vi "Wait.vi"(8 "Error In":errorcluster, 9 "timeout in ms (-1)":i32=-1, 11 "Init Waiter in":refnum<class "Init Waiter.lvclass">) -> (0 "Error Out":errorcluster, 1 "timed out?":bool)   [LabVIEW 2020, in "Panel.lvlib" / "Init Waiter.lvclass"]
doc: "Waits for the Panel to be initialized.\n<B>Init Waiter In:</B> Init Waiter to wait on\n<B>timeout in ms (-1):</B> Time to wait before timing out.\n<B>Error In:</B> Describes error conditions that occur before this node runs.\n\n<B>timed out?:</B> Indicates if the operation timed out.\n<B>Error Out:</B> Contains error information.\n----\nPlease see the following web address for additional documentation and tutorial information:\nhttp://www.mooregoodideas.com/mgi-panel-manager/\n\nAuthor: Derek Trepanier\n\nCopyright (c) 2018, Moore Good Ideas, Inc.\n\nAll rights reserved.\n\nRedistribution and use in source and binary forms, with or without modification, are permitted provided that the following conditions are met:\n\n * Redistributions of source code must retain the above copyright notice, this list of conditions and the following disclaimer.\n * Redistributions in binary form must reproduce the above copyright notice, this list of conditions and the following disclaimer in the documentation and/or other materials provided with the distribution.\n * Neither the name of Moore Good Ideas, Inc. nor the names of its contributors may be used to endorse or promote products derived from this software without specific prior written permission.\n\nTHIS SOFTWARE IS PROVIDED BY THE COPYRIGHT HOLDERS AND CONTRIBUTORS \"AS IS\" AND ANY EXPRESS OR IMPLIED WARRANTIES, INCLUDING, BUT NOT LIMITED TO, THE IMPLIED WARRANTIES OF MERCHANTABILITY AND FITNESS FOR A PARTICULAR PURPOSE ARE DISCLAIMED. IN NO EVENT SHALL THE COPYRIGHT OWNER OR CONTRIBUTORS BE LIABLE FOR ANY DIRECT, INDIRECT, INCIDENTAL, SPECIAL, EXEMPLARY, OR CONSEQUENTIAL DAMAGES (INCLUDING, BUT NOT LIMITED TO, PROCUREMENT OF SUBSTITUTE GOODS OR SERVICES; LOSS OF USE, DATA, OR PROFITS; OR BUSINESS INTERRUPTION) HOWEVER CAUSED AND ON ANY THEORY OF LIABILITY, WHETHER IN CONTRACT, STRICT LIABILITY, OR TORT (INCLUDING NEGLIGENCE OR OTHERWISE) ARISING IN ANY WAY OUT OF THE USE OF THIS SOFTWARE, EVEN IF ADVISED OF THE POSSIBILITY OF SUCH DAMAGE."
uses:
  <vilib>/MGI/Panel Manager/Panel/Init Waiter/Init Waiter.lvclass
  <vilib>/MGI/Panel Manager/Panel/Init Waiter/Init Waiter.lvclass/Init Waiter.ctl
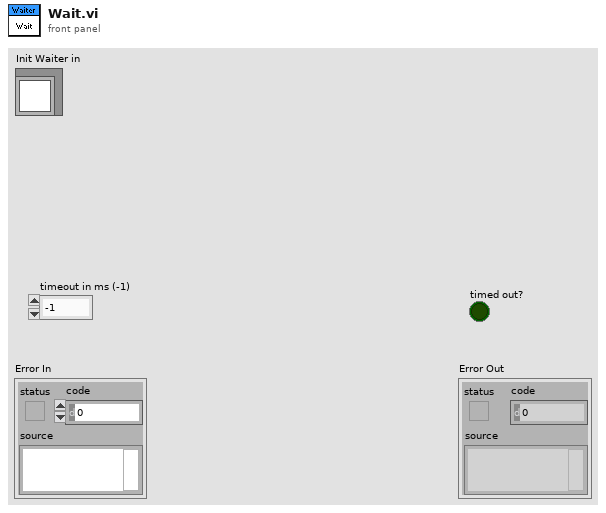
[diagram p1: front panel]
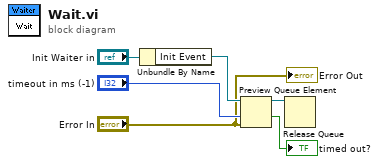
[diagram p0: block diagram]
diagram:
  n1 = Unbundle By Name("Init Waiter in") -> ("Init Event"=w5:refnum<queue>)
  n2 = Preview Queue Element(queue=w5, timeout in ms (-1)="timeout in ms (-1)", error in (no error)="Error In") -> (queue out=w1:refnum<queue>, timed out?=→"timed out?":bool)  [unwired: 2 out]
  n3 = Release Queue(queue=w1) -> ()  [unwired: 2 in, 3 out]
  "Error Out" <- "Error In"
